vi "Test Pixel Format.vi"(11 "Test Case In":refnum<class "Test.Camera.lvclass">) -> (0 "error out":errorcluster, 3 "Test Case Out":refnum<class "Test.Camera.lvclass">)   [LabVIEW 2020, in "Test.Camera.lvclass"]
uses:
  Test.Camera.lvclass
  C:/Program Files (x86)/National Instruments/LabVIEW 2020/vi.lib/Astemes/LUnit/Test Case.lvclass
  g_industrial_cam/Camera/Camera.lvclass/Camera.ctl
  <vilib>/Astemes/LUnit/Test Case.lvclass/Test Case.ctl
  011763c1-b056-4f54-ba36-7d1a9c65cae9.vi
  46839bd5-792c-4954-bd64-c3adb24b1d35.vi
  Get Alternative List Value.vi/469305e1-309a-4f6a-b6f2-863a5691b531.vi
  g_industrial_cam/Camera/GetSetPixelFormat.vi
  <vilib>/Astemes/LUnit/Core/LUnit Test Case/Private/Append Pass Result.vi
  <vilib>/Astemes/LUnit/Core/LUnit Test Case/Private/Append Fail Result.vi
  46839bd5-792c-4954-bd64-c3adb24b1d35.vi/9c5d11cd-9439-4240-a1ee-d9baace9c924.vi
  Get Alternative List Value.vi/469305e1-309a-4f6a-b6f2-863a5691b531.vi/544dbb3f-0ef1-42b7-8881-2db6294bd381.vi
  <vilib>/Astemes/LUnit/Core/LUnit Test Case/Private/Run In UI.vi
  <vilib>/Utility/error.llb/Clear Errors.vi
  g_industrial_cam/Camera/Check Not Disconnected.vi
  <vilib>/Utility/error.llb/Error Cluster From Error Code.vi
  <vilib>/Comparison/Equal/Equal Functor/Equal Functor.lvclass
  Test.Camera.lvclass/Test.Camera.ctl
  g_industrial_cam/Camera/Camera.lvclass
  <vilib>/Astemes/LUnit/Test Case.lvclass
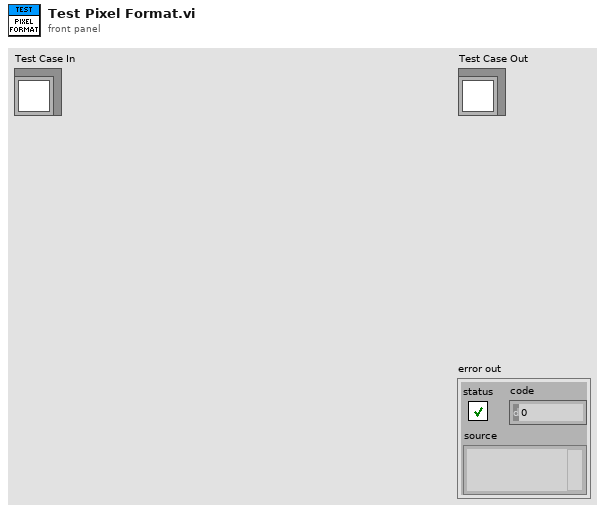
[diagram p1: front panel]
types:
  T1 = cluster{"Pixel Formats":string[], "Pixel Format":string}
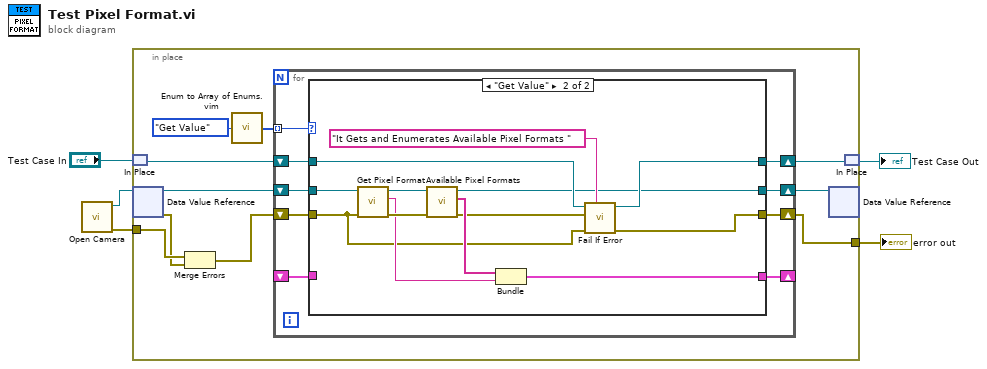
[diagram p0: block diagram]
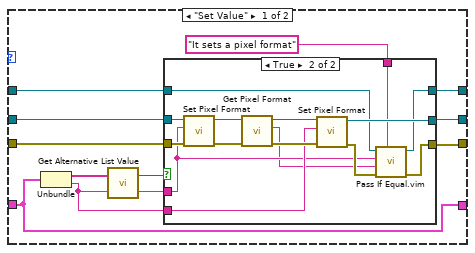
[diagram p2: hidden frame]
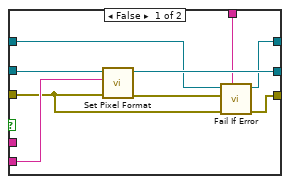
[diagram p3: hidden frame]
diagram:
  n1 = call "Open Camera.vi"() -> ("error out"=w5:errorcluster, "Camera"=w4:refnum<data-value>)  [unwired: 10 in]
  n2 = in-place {
    in-place-border: w5 -> [w15]
    in-place-border: [w6] -> w1
    n3 = in-place-match #1("Test Case In") -> (w11:refnum<class "Test.Camera.lvclass">)
    n4 = in-place-dvr #2(w4) -> (w14:refnum<class "Camera.lvclass">, w13:errorcluster)
    n5 = Merge Errors(w15, w13) -> (w12:errorcluster)
    n6 = call "Enum to Array of Enums.vim"("enum"=enum16{"Get Value", "Set Value"}."Get Value") -> ("array of enums"=w9:enum16{"Get Value", "Set Value"}[])
    n7 = for {
      shift-right: [w20] -> w8
      shift-left: w11 -> [w22]
      tunnel: w9 -> [w21] mode=indexing
      shift-right: [w19] -> w6
      shift-left: w12 -> [w23]
      shift-right: [w18] -> _
      shift-left: _ -> [w17]
      shift-right: [w16] -> w7
      shift-left: w14 -> [w24]
      n8 = case shown="\"Get Value\"" w21 {
        tunnel: w24 -> [w35 w73]
        tunnel: w23 -> [w32 w66]
        tunnel: w22 -> [w34 w72]
        tunnel: [w28 w65] -> w20
        tunnel: [w27 w64] -> w19
        tunnel: [w26 w63] -> w18
        tunnel: w17 -> [w26 _]
        tunnel: [w25 w61] -> w16
        frame "Set Value" {
          n9 = Unbundle(w26) -> ("Pixel Formats"=w36:string[], "Pixel Format"=w29:string)
          n10 = call "Get Alternative List Value.vi"("Current Value"=w29, "List in"=w36) -> ("Altenative Value"=w30:string, "Alternative Available"=w31:bool)
          n11 = case shown="True" w31 {
            tunnel: [w45 w56] -> w25
            tunnel: [w38 w46] -> w27
            tunnel: w35 -> [w42 w55]
            tunnel: w34 -> [w41 w54]
            tunnel: "It sets a pixel format" ("Description") -> [w40 w53]
            tunnel: w32 -> [w37 w51]
            tunnel: w30 -> [_ w49]
            tunnel: w29 -> [w43 w50]
            tunnel: [w39 w47] -> w28
            frame False {
              n12 = call "Set Pixel Format.vi"("error in (no error)"=w37, "Pixel Format"=w43, "Camera in"=w42) -> ("error out"=w44:errorcluster, "Camera"=w45:refnum<class "Camera.lvclass">)  [unwired: 7 in]
              n13 = call <vilib>:"Fail If Error.vi"("Description"=w40, "error in (no error)"=w37, "Assert error"=w44, "LUnit Test Case In"=w41) -> ("error out"=w38:errorcluster, "LUnit Test Case Out"=w39:refnum<class "Test.Camera.lvclass">)  [unwired: 6 in]
            }
            frame True {
              n14 = call "Set Pixel Format.vi"("error in (no error)"=w51, "Pixel Format"=w49, "Camera in"=w55) -> ("error out"=w58:errorcluster, "Camera"=w60:refnum<class "Camera.lvclass">)  [unwired: 7 in]
              n15 = call "Get Pixel Format.vi"("error in (no error)"=w58, "Camera in"=w60) -> ("error out"=w57:errorcluster, "Pixel Format"=w48:string, "Camera"=w59:refnum<class "Camera.lvclass">)  [unwired: 7 in]
              n16 = call "Set Pixel Format.vi"("error in (no error)"=w57, "Pixel Format"=w50, "Camera in"=w59) -> ("error out"=w52:errorcluster, "Camera"=w56:refnum<class "Camera.lvclass">)  [unwired: 7 in]
              n17 = call "Pass If Equal.vim"("Description"=w53, "error in (no error)"=w52, "Actual"=w48, "Expected"=w49, "LUnit Test Case In"=w54) -> ("error out"=w46:errorcluster, "LUnit Test Case Out"=w47:refnum<class "Test.Camera.lvclass">)  [unwired: 5 in]
            }
          }
        }
        frame "Get Value" {
          n18 = call "Get Pixel Format.vi"("error in (no error)"=w66, "Camera in"=w73) -> ("error out"=w71:errorcluster, "Pixel Format"=w70:string, "Camera"=w62:refnum<class "Camera.lvclass">)  [unwired: 7 in]
          n19 = call "Available Pixel Formats.vi"("error in (no error)"=w71, "Camera in"=w62) -> ("error out"=w67:errorcluster, "Pixel Formats"=w69:string[], "Camera"=w61:refnum<class "Camera.lvclass">)  [unwired: 7 in]
          n20 = Bundle("Pixel Formats"=w69, "Pixel Format"=w70) -> (w63:T1)  [unwired: 1 in]
          n21 = call <vilib>:"Fail If Error.vi"("Description"="It Gets and Enumerates Available Pixel Formats ", "error in (no error)"=w66, "Assert error"=w67, "LUnit Test Case In"=w72) -> ("error out"=w64:errorcluster, "LUnit Test Case Out"=w65:refnum<class "Test.Camera.lvclass">)  [unwired: 6 in]
        }
      }
    }
    n22 = in-place-dvr #2(w7) -> ()  [unwired: 2 out]
    n23 = in-place-match #1(w8) -> (→"Test Case Out":refnum<class "Test.Camera.lvclass">)
  }
  "error out" <- w1
